vi "enumerateStaticDependencies.vi"(8 "error in (no error)":errorcluster, 11 "Measurement.WavelengthSweeping":refnum<class "Measurement.WavelengthSweeping.lvclass">) -> (0 "error out":errorcluster, 2 "Static Dependencies":refnum<class "Dependency.lvclass">[](array[class]), 3 "Measurement.WavelengthSweeping out":refnum<class "Measurement.WavelengthSweeping.lvclass">)   [LabVIEW 2019, in "Measurement.WavelengthSweeping.lvclass"]
doc: "JKI State Machine Objects (SMO) 1.3.0.56\nJKI - JKI\nCopyright (c) 2017, JKI"
uses:
  Measurement.WavelengthSweeping.lvclass
  <vilib>/JKI/JKI SMO/Dependency/Dependency.lvclass
  SMU/SMU.lvclass
  C:/Program Files (x86)/National Instruments/LabVIEW 2019/vi.lib/JKI/JKI SMO/SMO/SMO.lvclass
  LIA/LIA.lvclass
  OPM/OPM.lvclass
  OPA/OPA.lvclass
  Typedefs/Dependencies--Cluster.ctl
  MC/MC.lvclass
  Device/Device.lvclass
  Measurement/Measurement.lvclass
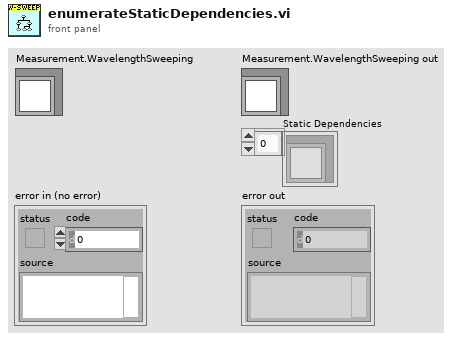
[diagram p1: front panel]
types:
  T1 = typedef "Measurement.WavelengthSweeping.lvclass/Dependencies--Cluster.ctl" = cluster{"SMU":refnum<class "SMU.lvclass">, "LIA":refnum<class "LIA.lvclass">, "OPM":refnum<class "OPM.lvclass">, "OPA":refnum<class "OPA.lvclass">, "MC":refnum<class "MC.lvclass">}
  T2 = typedef "Measurement.WavelengthSweeping.lvclass/Configuration--Cluster.ctl" = cluster{"Measurement.Type":T3, "Hardware":T4, "Measurement":T15}
  T3 = typedef "Measurement.lvclass/Measurement.Type--Enum.ctl" = enum16{"Free", "I/V Curve", "Wavelength sweeping", "Photocurrent mapping"}
  T4 = typedef "Measurement.WavelengthSweeping.lvclass/Configuration.Hardware--Cluster.ctl" = cluster{"SMU":T5, "LIA":T7, "OPM":T9, "OPA":T11, "MC":T13}
  T5 = typedef "Measurement.lvclass/Configuration.SMU--Cluster.ctl" = cluster{"Enable":bool, "SMU Model":string, "Configuration":T6}
  T6 = typedef "SMU.lvclass/Configuration--Cluster.ctl" = cluster{"VISA Resource":string, "Channel":string}
  T7 = typedef "Measurement.lvclass/Configuration.LIA--Cluster.ctl" = cluster{"Enable":bool, "LIA Model":string, "Configuration":T8}
  T8 = typedef "LIA.lvclass/Configuration--Cluster.ctl" = cluster{"VISA Resource":string}
  T9 = typedef "Measurement.lvclass/Configuration.OPM--Cluster.ctl" = cluster{"Enable":bool, "OPM Model":string, "Configuration":T10}
  T10 = typedef "OPM.lvclass/Configuration--Cluster.ctl" = cluster{"VISA Resource":string}
  T11 = typedef "Measurement.lvclass/Configuration.OPA--Cluster.ctl" = cluster{"Enable":bool, "OPA Model":string, "Configuration":T12}
  T12 = typedef "OPA.lvclass/Configuration--Cluster.ctl" = cluster{"Serial Number":string}
  T13 = typedef "Measurement.lvclass/Configuration.MC--Cluster.ctl" = cluster{"Enable":bool, "MC Model":string, "Configuration":T14}
  T14 = typedef "MC.lvclass/Configuration--Cluster.ctl" = cluster{"VISA Resource":string}
  T15 = typedef "Measurement.WavelengthSweeping.lvclass/Configuration.Measurement--Cluster.ctl" = cluster{"SMU Voltage, V":dbl, "Start wavelength, nm":dbl, "Stop wavelength, nm":dbl, "Scan resolution, nm":dbl, "Number or points":u16, "Integration time, sec":dbl, "Delay time, ms":u16, "Accumulation":u16, "Wavelength offset, nm":dbl}
  T16 = cluster{"SMU":refnum<class "SMU.lvclass">, "LIA":refnum<class "LIA.lvclass">, "OPM":refnum<class "OPM.lvclass">, "OPA":refnum<class "OPA.lvclass">, "MC":refnum<class "MC.lvclass">}
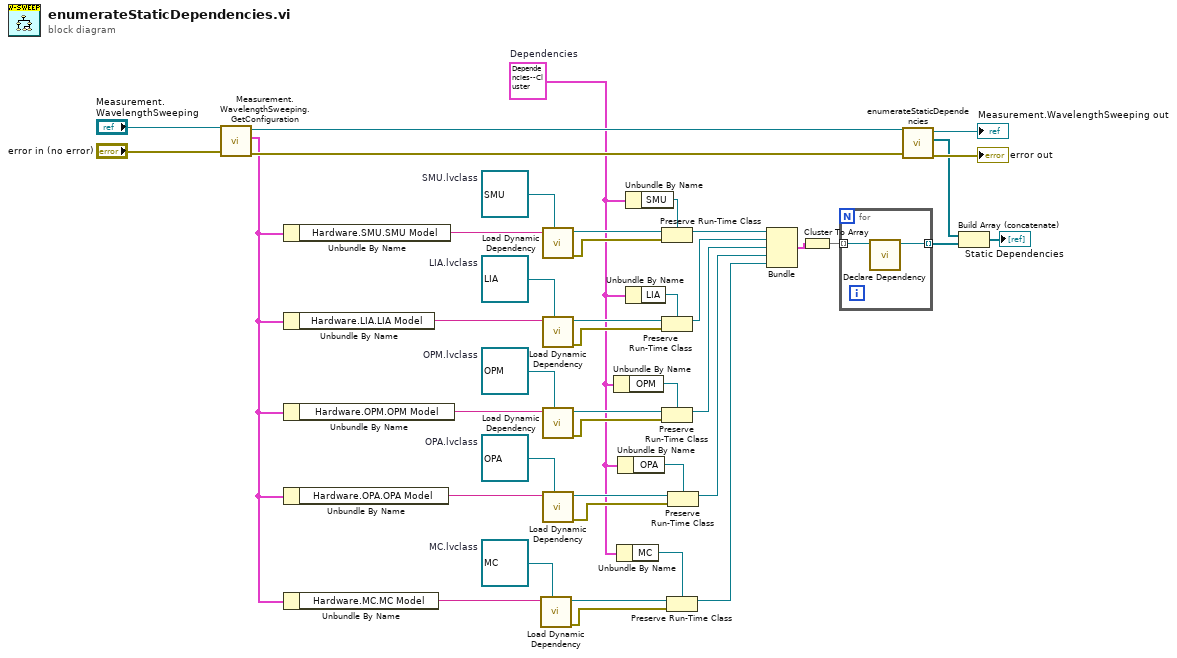
[diagram p0: block diagram]
diagram:
  w8 = refnum<class "MC.lvclass"> refnum  # MC.lvclass
  w2 = T1 {"SMU"=refnum, "LIA"=refnum, "OPM"=refnum, "OPA"=refnum, "MC"=refnum}  # Dependencies
  w17 = refnum<class "OPA.lvclass"> refnum  # OPA.lvclass
  w26 = refnum<class "OPM.lvclass"> refnum  # OPM.lvclass
  w33 = refnum<class "LIA.lvclass"> refnum  # LIA.lvclass
  w40 = refnum<class "SMU.lvclass"> refnum  # SMU.lvclass
  n1 = call "Measurement.WavelengthSweeping.GetConfiguration.vi"("error in (no error)"="error in (no error)", "Measurement.WavelengthSweeping"="Measurement.WavelengthSweeping") -> ("error out"=w12:errorcluster, "Configuration"=w7:T2, "Measurement.WavelengthSweeping out"=w13:refnum<class "Measurement.WavelengthSweeping.lvclass">)  [unwired: 7 in]
  n2 = Unbundle By Name(w7) -> ("Hardware.SMU.SMU Model"=w41:string)
  n3 = Unbundle By Name(w7) -> ("Hardware.LIA.LIA Model"=w28:string)
  n4 = Unbundle By Name(w7) -> ("Hardware.OPM.OPM Model"=w27:string)
  n5 = Unbundle By Name(w7) -> ("Hardware.OPA.OPA Model"=w19:string)
  n6 = Unbundle By Name(w7) -> ("Hardware.MC.MC Model"=w6:string)
  n7 = call "Load Dynamic Dependency.vi"("SMO in"=w8, "Class Name"=w6) -> ("error out"=w3:errorcluster, "SMO out"=w4:refnum<class "MC.lvclass">)  [unwired: 8 in]
  n8 = call "Load Dynamic Dependency.vi"("SMO in"=w40, "Class Name"=w41) -> ("error out"=w37:errorcluster, "SMO out"=w38:refnum<class "SMU.lvclass">)  [unwired: 8 in]
  n9 = call "Load Dynamic Dependency.vi"("SMO in"=w33, "Class Name"=w28) -> ("error out"=w30:errorcluster, "SMO out"=w31:refnum<class "LIA.lvclass">)  [unwired: 8 in]
  n10 = call "Load Dynamic Dependency.vi"("SMO in"=w26, "Class Name"=w27) -> ("error out"=w24:errorcluster, "SMO out"=w25:refnum<class "OPM.lvclass">)  [unwired: 8 in]
  n11 = call "Load Dynamic Dependency.vi"("SMO in"=w17, "Class Name"=w19) -> ("error out"=w21:errorcluster, "SMO out"=w20:refnum<class "OPA.lvclass">)  [unwired: 8 in]
  n12 = Unbundle By Name(w2) -> ("OPM"=w23:refnum<class "OPM.lvclass">)
  n13 = Unbundle By Name(w2) -> ("MC"=w5:refnum<class "MC.lvclass">)
  n14 = Unbundle By Name(w2) -> ("OPA"=w18:refnum<class "OPA.lvclass">)
  n15 = Unbundle By Name(w2) -> ("SMU"=w39:refnum<class "SMU.lvclass">)
  n16 = Unbundle By Name(w2) -> ("LIA"=w32:refnum<class "LIA.lvclass">)
  n17 = Preserve Run-Time Class(object in=w38, error in=w37, 2:w39) -> (object out=w36:refnum<class "SMU.lvclass">)  [unwired: 1 out]
  n18 = Preserve Run-Time Class(object in=w31, error in=w30, 2:w32) -> (object out=w29:refnum<class "LIA.lvclass">)  [unwired: 1 out]
  n19 = Preserve Run-Time Class(object in=w25, error in=w24, 2:w23) -> (object out=w22:refnum<class "OPM.lvclass">)  [unwired: 1 out]
  n20 = Preserve Run-Time Class(object in=w4, error in=w3, 2:w5) -> (object out=w1:refnum<class "MC.lvclass">)  [unwired: 1 out]
  n21 = Preserve Run-Time Class(object in=w20, error in=w21, 2:w18) -> (object out=w16:refnum<class "OPA.lvclass">)  [unwired: 1 out]
  n22 = Bundle("SMU"=w36, "LIA"=w29, "OPM"=w22, "OPA"=w16, "MC"=w1) -> (w35:T16)  [unwired: 1 in]
  n23 = Cluster To Array(cluster=w35) -> (array=w34:refnum<class "Device.lvclass">[])
  n24 = for {
    tunnel: [w45] -> w11 mode=indexing
    tunnel: w34 -> [w44] mode=indexing
    n25 = call <vilib>:"Declare Dependency.vi"("Type"=w44) -> ("Dependency out"=w45:refnum<class "Dependency.lvclass">)  [unwired: 9 in, 1 out]
  }
  n26 = call-parent "enumerateStaticDependencies.vi"("error in (no error)"=w12, "SMO"=w13) -> ("error out"=→"error out":errorcluster, "Static Dependencies"=w10:refnum<class "Dependency.lvclass">[], "SMO out"=→"Measurement.WavelengthSweeping out":refnum<class "Measurement.WavelengthSweeping.lvclass">)  [unwired: 7 in]
  n27 = Build Array (concatenate)(w10, w11) -> (→"Static Dependencies":refnum<class "Dependency.lvclass">[])
